vi "Angle_To_Volt.vi"(0 "Angulo IN":dbl min=-30.0 max=30.0, 11 "Error In":errorcluster) -> (4 "Voltaje OUT":dbl, 15 "Error Out":errorcluster)   [LabVIEW 2016]
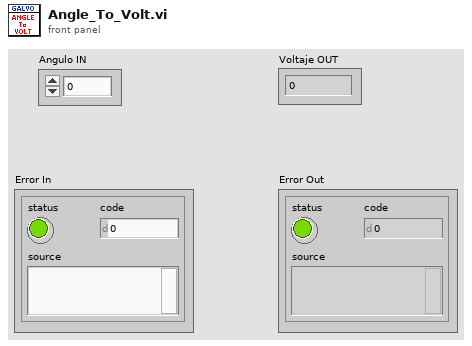
[diagram p1: front panel]
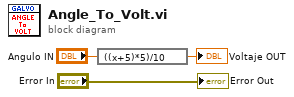
[diagram p0: block diagram]
diagram:
  n1 = expression code="((x+5)*5)/10"("Angulo IN") -> (→"Voltaje OUT":dbl)
  "Error Out" <- "Error In"
